vi "DPT Create Header File.vi"(8 "Supply Voltage:":string, 9 "Test_Type:":string, 10 "Output Dryer Information":T1={"Dryer Type"="", "TR Number"="", "Lab ID"="", "Output Stream Header"=[], "Stream Data Output"=[], "2015 Array"=[], "Dryer Test Data"=[], "Off Mode Array"=[], "Calibration Array"=[], "File Initialization Array"=[], "Load Run Number"="", "Model:"="", "Serial Number:"="", "Build:"="", "Test_Title Per TR:"="", "Ambient Temp SetPoint:"="", "Washer Water \nTemperature ( 60 ± 5°F ):"="", "Frequency:"="", "Dryness Setting:"="", "Heat Setting:"="", "Ambient RH:"="", "Drying Cycle:"="", "Exhaust:"="", "Comments:"="", "Technician:"="", "Engineer:"="", "Water Hardness (PPM)"="", "Empty Dryer Cold Weight"="", "Date:"="", "Version:"="", "Computer:"="", "Load Type"="", "Nominal Load  Weight"="", "Weights Out"={"Measured IMC"=7.0, "Actual RMC"=7.0, "RMC (Desired)"=100.0, "Bone Dry Wt(lbs)"=7.0, "Tolerance(%)"=5.0}, "Test Station:"="1A", "Heat Setting:"="1A", "Dryness Setting:"="", "Frequency:"="", "Water Hardness (PPM)"="", "Washer Water \nTemperature ( 60 ± 5°F )"="", "Flow Computer Info Baro,BTUF,u,Z"=[], "Filename"="", "Analog Voltage Data"=[]} {"Weights Out"."Tolerance(%)" format="%0#_6g"; "Weights Out"."Bone Dry Wt(lbs)" format="%03_6g"; "Weights Out"."RMC (Desired)" format="%0#_6g"; "Weights Out"."Actual RMC" format="%03_6g"; "Weights Out"."Measured IMC" format="%0#_6g"}, 11 "Flow Computer Info Baro,BTUF,u,Z":string[][](array[string])) -> (3 "Array":string[][](array[string]))   [LabVIEW 2016, in "File Setup.lvlib"]
uses:
  File Setup.lvlib
  Type Definition/DPT Output Dryer Information.ctl
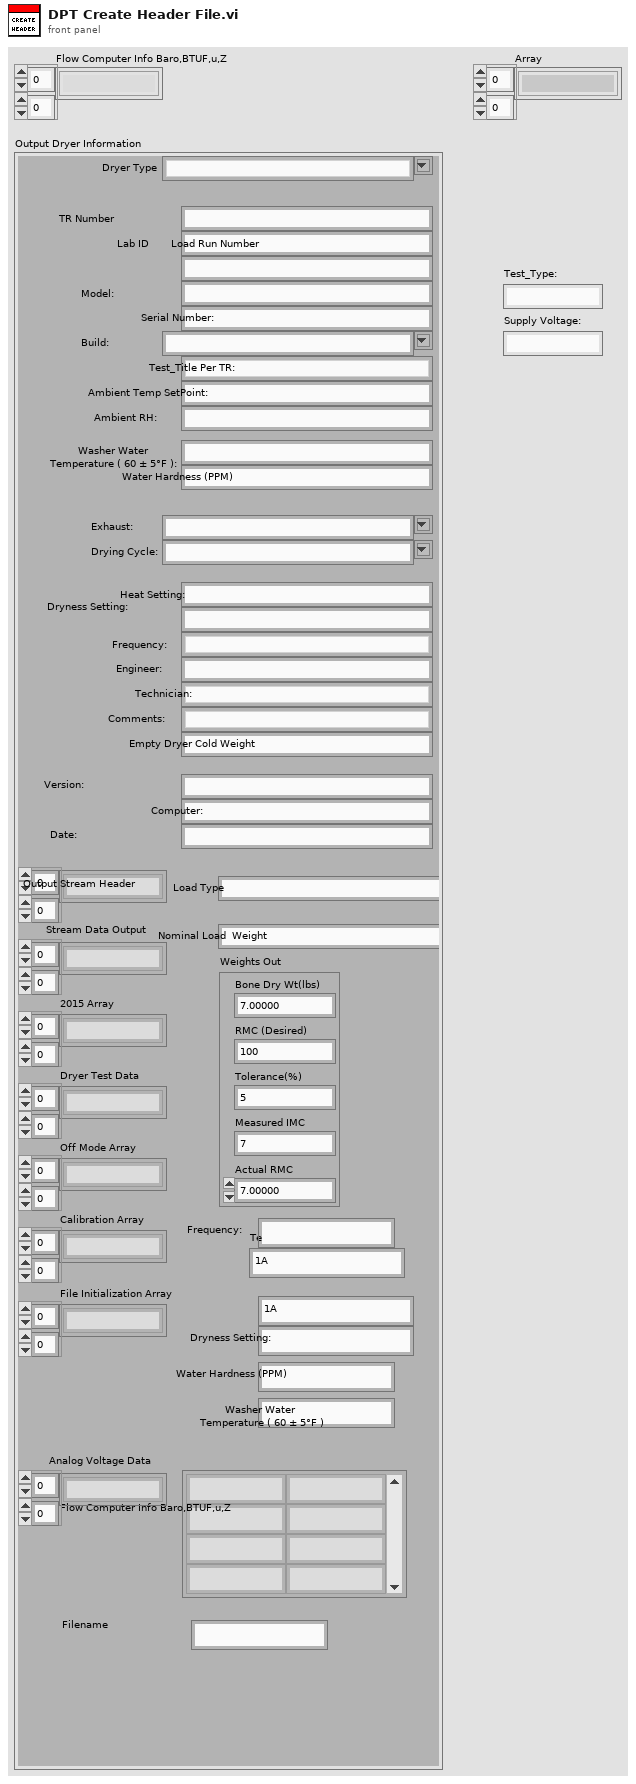
[diagram p1: front panel]
types:
  T1 = typedef "File Setup.lvlib/DPT Output Dryer Information.ctl" = cluster{"Dryer Type":string, "TR Number":string, "Lab ID":string, "Output Stream Header":string[][], "Stream Data Output":string[][], "2015 Array":string[][], "Dryer Test Data":string[][], "Off Mode Array":string[][], "Calibration Array":string[][], "File Initialization Array":string[][], "Load Run Number":string, "Model:":string, "Serial Number:":string, "Build:":string, "Test_Title Per TR:":string, "Ambient Temp SetPoint:":string, "Washer Water \nTemperature ( 60 ± 5°F ):":string, "Frequency:":string, "Dryness Setting:":string, "Heat Setting:":string, "Ambient RH:":string, "Drying Cycle:":string, "Exhaust:":string, "Comments:":string, "Technician:":string, "Engineer:":string, "Water Hardness (PPM)":string, "Empty Dryer Cold Weight":string, "Date:":string, "Version:":string, "Computer:":string, "Load Type":string, "Nominal Load  Weight":string, "Weights Out":cluster{"Measured IMC":dbl, "Actual RMC":dbl, "RMC (Desired)":dbl, "Bone Dry Wt(lbs)":dbl, "Tolerance(%)":dbl}, "Test Station:":string, "Heat Setting:":string, "Dryness Setting:":string, "Frequency:":string, "Water Hardness (PPM)":string, "Washer Water \nTemperature ( 60 ± 5°F )":string, "Flow Computer Info Baro,BTUF,u,Z":string[][], "Filename":string, "Analog Voltage Data":string[][]}
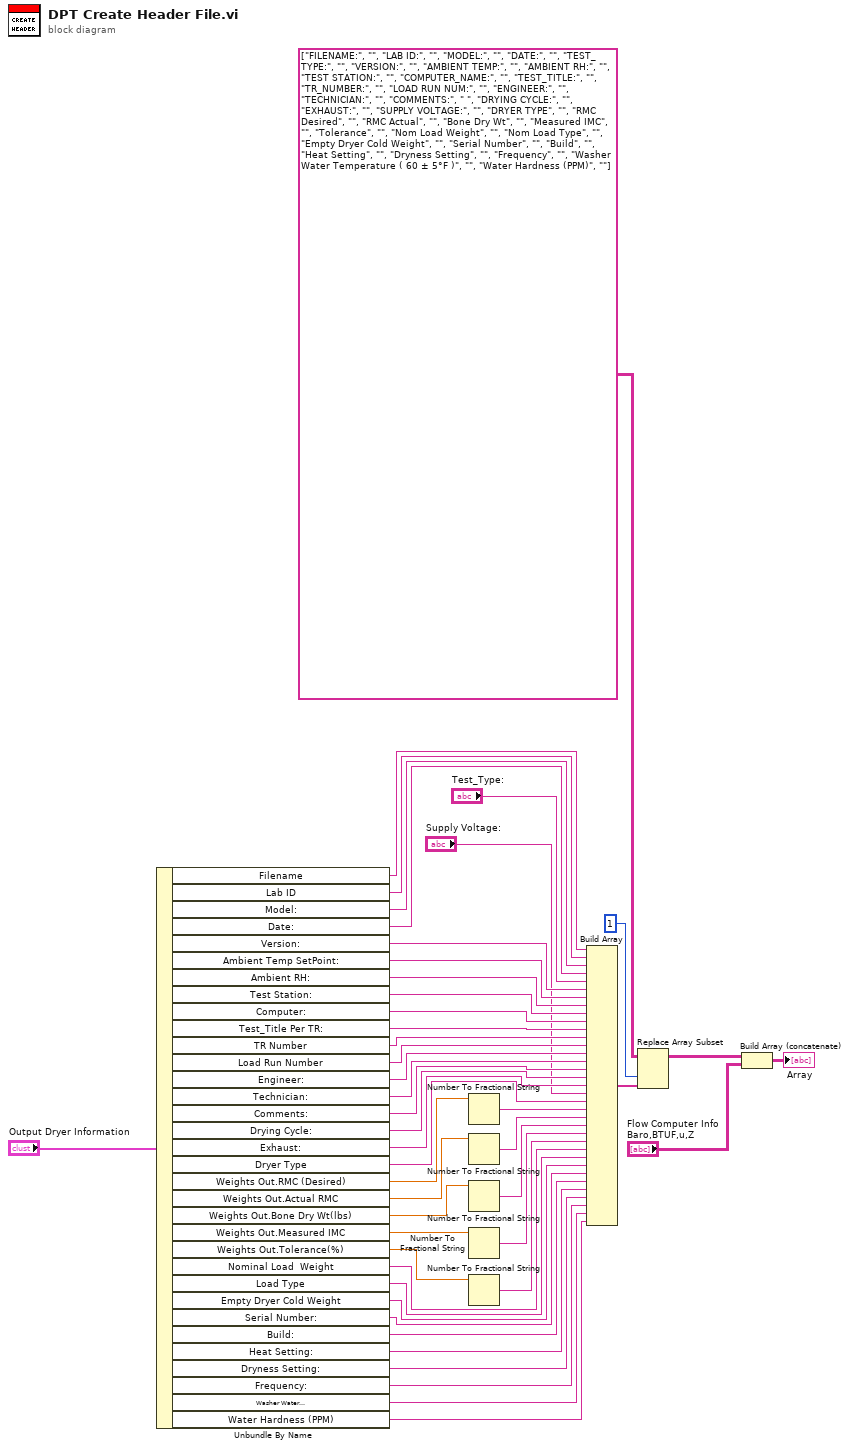
[diagram p0: block diagram]
diagram:
  n1 = Unbundle By Name("Output Dryer Information") -> ("Filename"=w30:string, "Lab ID"=w29:string, "Model:"=w28:string, "Date:"=w27:string, "Version:"=w25:string, "Ambient Temp SetPoint:"=w24:string, "Ambient RH:"=w23:string, "Test Station:"=w22:string, "Computer:"=w21:string, "Test_Title Per TR:"=w20:string, "TR Number"=w19:string, "Load Run Number"=w18:string, "Engineer:"=w17:string, "Technician:"=w16:string, "Comments:"=w15:string, "Drying Cycle:"=w14:string, "Exhaust:"=w13:string, "Dryer Type"=w11:string, "Weights Out.RMC (Desired)"=w34:dbl, "Weights Out.Actual RMC"=w35:dbl, "Weights Out.Bone Dry Wt(lbs)"=w36:dbl, "Weights Out.Measured IMC"=w37:dbl, "Weights Out.Tolerance(%)"=w42:dbl, "Nominal Load  Weight"=w10:string, "Load Type"=w9:string, "Empty Dryer Cold Weight"=w8:string, "Serial Number:"=w7:string, "Build:"=w6:string, "Heat Setting:"=w5:string, "Dryness Setting:"=w4:string, "Frequency:"=w3:string, "Washer Water \nTemperature ( 60 ± 5°F ):"=w2:string, "Water Hardness (PPM)"=w1:string)
  n2 = Number To Fractional String(number=w34) -> (F-format string=w38:string)  [unwired: 3 in]
  n3 = Number To Fractional String(number=w35) -> (F-format string=w39:string)  [unwired: 3 in]
  n4 = Number To Fractional String(number=w36) -> (F-format string=w40:string)  [unwired: 3 in]
  n5 = Number To Fractional String(number=w37) -> (F-format string=w41:string)  [unwired: 3 in]
  n6 = Number To Fractional String(number=w42) -> (F-format string=w43:string)  [unwired: 3 in]
  n7 = Build Array(w30, w29, w28, w27, "Test_Type:", w25, w24, w23, w22, w21, w20, w19, w18, w17, w16, w15, w14, w13, "Supply Voltage:", w11, w38, w39, w40, w41, w43, w10, w9, w8, w7, w6, w5, w4, w3, w2, w1) -> (w32:string[])
  n8 = Replace Array Subset(array=string[][] [["FILENAME:", ""], ["LAB ID:", ""], ["MODEL:", ""], ["DATE:", ""], ["TEST_TYPE:", ""], ["VERSION:", ""], ["AMBIENT TEMP:", ""], ["AMBIENT RH:", ""], ["TEST STATION:", ""], ["COMPUTER_NAME:", ""], ["TEST_TITLE:", ""], ["TR_NUMBER:", ""], ["LOAD RUN NUM:", ""], ["ENGINEER:", ""], ["TECHNICIAN:", ""], ["COMMENTS:", " "], ["DRYING CYCLE:", ""], ["EXHAUST:", ""], ["SUPPLY VOLTAGE:", ""], ["DRYER TYPE", ""], ["RMC Desired", ""], ["RMC Actual", ""], ["Bone Dry Wt", ""], ["Measured IMC", ""], ["Tolerance", ""], ["Nom Load Weight", ""], ["Nom Load Type", ""], ["Empty Dryer Cold Weight", ""], ["Serial Number", ""], ["Build", ""], ["Heat Setting", ""], ["Dryness Setting", ""], ["Frequency", ""], ["Washer Water Temperature ( 60 ± 5°F )", ""], ["Water Hardness (PPM)", ""]], new element=w32, index (col)=1 ("disabled index (col)")) -> (w45:string[][])  [unwired: 1 in]
  n9 = Build Array (concatenate)(w45, "Flow Computer Info Baro,BTUF,u,Z") -> (→"Array":string[][])
